vi "InterfaceByViServer_Example1.vi"() -> ()   [LabVIEW 2019]
uses:
  Sub_class/Sub.lvclass
  Base_class/Base.lvclass
  Leaf_class/Leaf.lvclass
  Interface1_Interface/Interface1.lvclass
panel:
  out "String 3":string
  out "error out 3":errorcluster
  out "error out 2":errorcluster
  out "String 2":string
  out "String 1":string
  out "error out 1":errorcluster
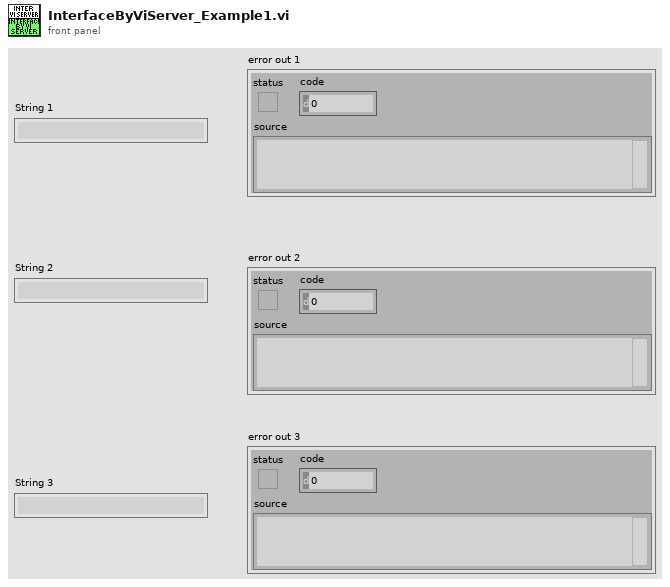
[diagram p1: front panel]
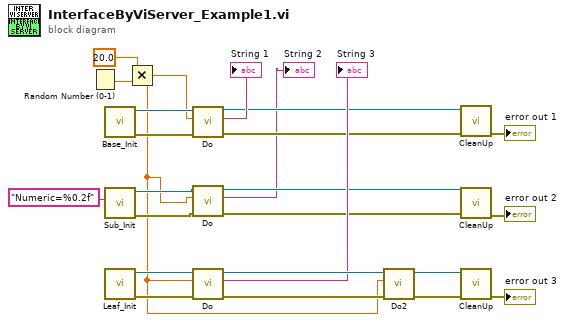
[diagram p0: block diagram]
diagram:
  n1 = Random Number (0-1)() -> (number: 0 to 1=w24:dbl)
  n2 = call "Base_Init.vi"() -> ("error out"=w14:errorcluster, "object out"=w15:refnum<class "Base.lvclass">)  [unwired: 10 in]
  n3 = call "Sub_Init.vi"("String"="Numeric=%0.2f") -> ("error out"=w5:errorcluster, "object out"=w6:refnum<class "Sub.lvclass">)  [unwired: 9 in]
  n4 = call "Leaf_Init.vi"() -> ("error out"=w21:errorcluster, "object out"=w20:refnum<class "Leaf.lvclass">)  [unwired: 10 in]
  n5 = Multiply(x=20.0, y=w24) -> (x*y=w1:dbl)
  n6 = call "Do.vi"("error in (no error)"=w14, "Numeric"=w1, "Interface In"=w15) -> ("error out"=w13:errorcluster, "String"=→"String 1":string, "Interface Out"=w12:refnum<class "Base.lvclass">)  [unwired: 6 in]
  n7 = call "Do.vi"("error in (no error)"=w5, "Numeric"=w1, "Interface In"=w6) -> ("error out"=w3:errorcluster, "String"=→"String 2":string, "Interface Out"=w4:refnum<class "Sub.lvclass">)  [unwired: 6 in]
  n8 = call "Do.vi"("error in (no error)"=w21, "Numeric"=w1, "Interface In"=w20) -> ("error out"=w8:errorcluster, "String"=→"String 3":string, "Interface Out"=w19:refnum<class "Leaf.lvclass">)  [unwired: 6 in]
  n9 = call "Do2.vi"("error in (no error)"=w8, "Numeric"=w1, "Interface In"=w19) -> ("error out"=w7:errorcluster, "Interface Out"=w9:refnum<class "Leaf.lvclass">)  [unwired: 6 in, 1 out]
  n10 = call-dynamic "CleanUp.vi"("error in (no error)"=w13, "object in"=w12) -> ("error out"=→"error out 1":errorcluster)  [unwired: 8 in, 1 out]
  n11 = call-dynamic "CleanUp.vi"("error in (no error)"=w3, "Object in"=w4) -> ("error out"=→"error out 2":errorcluster)  [unwired: 8 in, 1 out]
  n12 = call-dynamic "CleanUp.vi"("error in (no error)"=w7, "Object in"=w9) -> ("error out"=→"error out 3":errorcluster)  [unwired: 8 in, 1 out]
